vi "Temp_Read_Sub.vi"(0 "VISA Refnum in":refnum<visa-resource-name>, 1 "Setp":refnum<vi>, 2 "Numeric":i32, 3 "String":string, 5 "String to Write":string, 7 "Rate":refnum<vi>, 9 "String to Write 2":string, 11 "Ring Refnum":refnum<vi>, 12 "Ring Refnum 2":refnum<vi>, 13 "String to Write 4":string, 14 "String to Write 3":string) -> (4 "Temp":dbl caption="K" format="%.4g", 6 "dup VISA Session":refnum<visa-resource-name>)   [LabVIEW 2024]
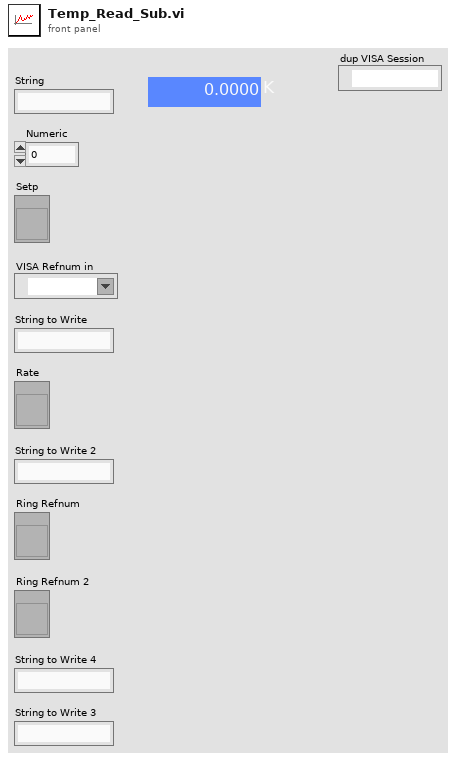
[diagram p1: front panel]
types:
  T1 = enum8{"Enabled", "Disabled", "Disabled and Grayed Out"}
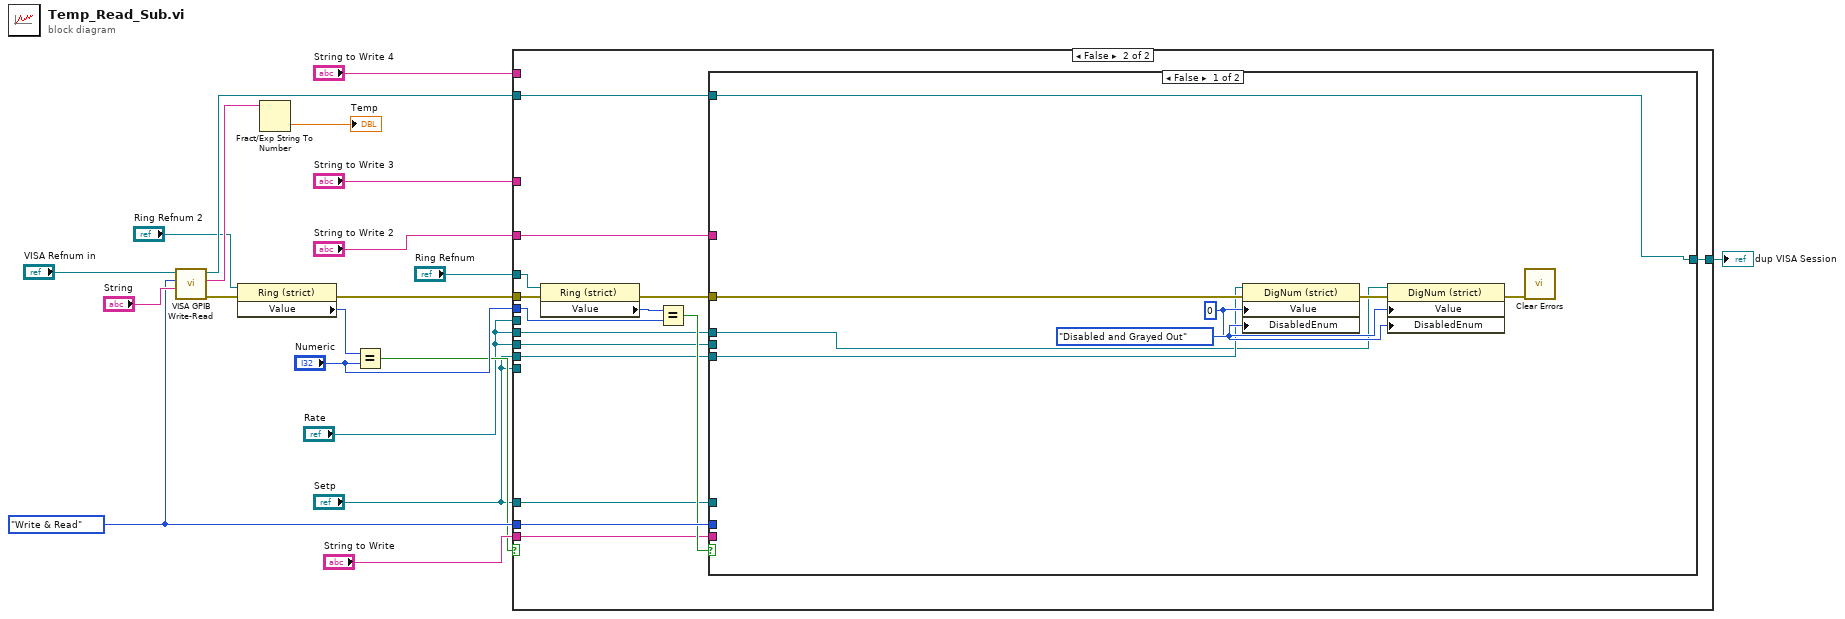
[diagram p0: block diagram]
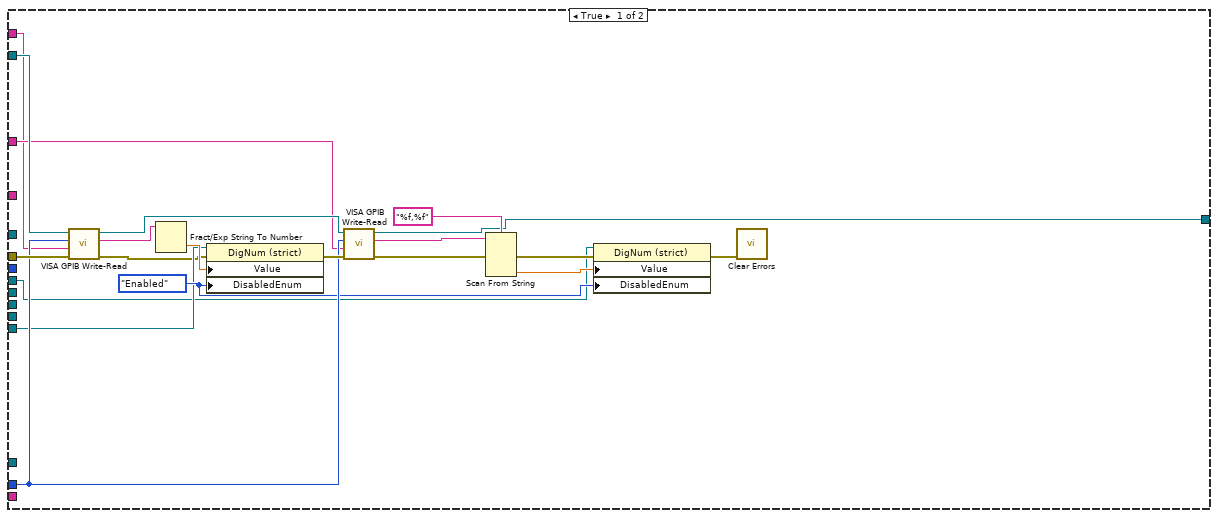
[diagram p2: hidden frame]
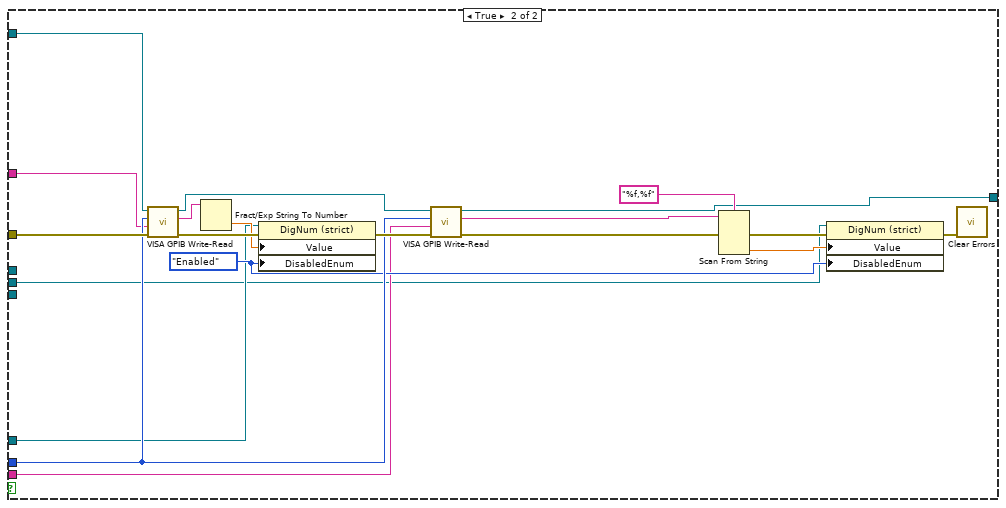
[diagram p3: hidden frame]
diagram:
  w12 = enum16{"Write", "Read", "Write & Read"}."Write & Read" ("Action")
  n1 = call "VISA GPIB Write-Read.vi"("Command"="String", "Action"=w12, "VISA resource name"="VISA Refnum in") -> ("error out"=w9:errorcluster, "String Returned"=w7:string, "dup VISA Session"=w13:refnum<visa-resource-name>)  [unwired: 5 in, 1 out]
  n2 = property on="Property Node" class="Ring (strict)"(reference="Ring Refnum 2", error in=w9) -> (error out=w2:errorcluster, "Value"=w10:u16)  [unwired: 1 out]
  n3 = Fract/Exp String To Number(string=w7) -> (number=→"Temp":dbl)  [unwired: 3 in, 1 out]
  n4 = Equal?(x=w10, y="Numeric") -> (x = y?=w11:bool)
  n5 = case shown="False" w11 {
    tunnel: w2 -> [w40 w53]
    tunnel: w12 -> [w34 w54]
    tunnel: w13 -> [w39 w55]
    tunnel: "Numeric" -> [_ w49]
    tunnel: "String to Write 3" -> [w27 _]
    tunnel: "String to Write 4" -> [w26 _]
    tunnel: "String to Write 2" -> [_ w48]
    tunnel: "String to Write" -> [_ w47]
    tunnel: "Setp" -> [w24 _]
    tunnel: "Rate" -> [w23 _]
    tunnel: "Setp" -> [_ w46]
    tunnel: "Rate" -> [_ w45]
    tunnel: "Setp" -> [_ w44]
    tunnel: "Rate" -> [_ w43]
    tunnel: "Ring Refnum" -> [_ w42]
    tunnel: [w21 w41] -> w1
    frame True {
      w29 = T1."Enabled" ("Disabled")
      n6 = call "VISA GPIB Write-Read.vi"("error in (no error)"=w40, "Command"=w26, "Action"=w34, "VISA resource name"=w39) -> ("error out"=w22:errorcluster, "String Returned"=w38:string, "dup VISA Session"=w35:refnum<visa-resource-name>)  [unwired: 4 in, 1 out]
      n7 = Fract/Exp String To Number(string=w38) -> (number=w37:dbl)  [unwired: 3 in, 1 out]
      n8 = property on="Property Node" class="DigNum (strict)"(reference=w24, error in=w22, "Value"=w37, "DisabledEnum"=w29) -> (error out=w36:errorcluster)  [unwired: 1 out]
      n9 = call "VISA GPIB Write-Read.vi"("error in (no error)"=w36, "Command"=w27, "Action"=w34, "VISA resource name"=w35) -> ("error out"=w33:errorcluster, "String Returned"=w32:string, "dup VISA Session"=w21:refnum<visa-resource-name>)  [unwired: 4 in, 1 out]
      n10 = Scan From String(format string="%f,%f", input string=w32, error in=w33) -> (error out=w30:errorcluster, output 2=w28:dbl)  [unwired: 4 in, 2 out]
      n11 = property on="Property Node" class="DigNum (strict)"(reference=w23, error in=w30, "Value"=w28, "DisabledEnum"=w29) -> (error out=w25:errorcluster)  [unwired: 1 out]
      n12 = call <vilib>:"Clear Errors.vi"("error in (no error)"=w25) -> ()  [unwired: 5 in, 2 out]
    }
    frame False {
      n13 = property on="Property Node" class="Ring (strict)"(reference=w42, error in=w53) -> (error out=w52:errorcluster, "Value"=w51:u16)  [unwired: 1 out]
      n14 = Equal?(x=w51, y=w49) -> (x = y?=w50:bool)
      n15 = case shown="False" w50 {
        tunnel: w52 -> [w63 w83]
        tunnel: w55 -> [w56 w82]
        tunnel: w54 -> [_ w76]
        tunnel: w48 -> [_ w69]
        tunnel: w47 -> [_ w68]
        tunnel: w46 -> [w58 _]
        tunnel: w45 -> [w57 _]
        tunnel: w44 -> [_ w66]
        tunnel: w43 -> [_ w65]
        tunnel: [w56 w64] -> w41
        frame False {
          w61 = T1."Disabled and Grayed Out" ("Disabled")
          w60 = 0
          n16 = property on="Property Node" class="DigNum (strict)"(reference=w58, error in=w63, "Value"=w60, "DisabledEnum"=w61) -> (error out=w62:errorcluster)  [unwired: 1 out]
          n17 = property on="Property Node" class="DigNum (strict)"(reference=w57, error in=w62, "Value"=w60, "DisabledEnum"=w61) -> (error out=w59:errorcluster)  [unwired: 1 out]
          n18 = call <vilib>:"Clear Errors.vi"("error in (no error)"=w59) -> ()  [unwired: 5 in, 2 out]
        }
        frame True {
          w71 = T1."Enabled" ("Disabled")
          n19 = call "VISA GPIB Write-Read.vi"("error in (no error)"=w83, "Command"=w69, "Action"=w76, "VISA resource name"=w82) -> ("error out"=w80:errorcluster, "String Returned"=w81:string, "dup VISA Session"=w77:refnum<visa-resource-name>)  [unwired: 4 in, 1 out]
          n20 = Fract/Exp String To Number(string=w81) -> (number=w79:dbl)  [unwired: 3 in, 1 out]
          n21 = property on="Property Node" class="DigNum (strict)"(reference=w66, error in=w80, "Value"=w79, "DisabledEnum"=w71) -> (error out=w78:errorcluster)  [unwired: 1 out]
          n22 = call "VISA GPIB Write-Read.vi"("error in (no error)"=w78, "Command"=w68, "Action"=w76, "VISA resource name"=w77) -> ("error out"=w75:errorcluster, "String Returned"=w74:string, "dup VISA Session"=w64:refnum<visa-resource-name>)  [unwired: 4 in, 1 out]
          n23 = Scan From String(format string="%f,%f", input string=w74, error in=w75) -> (error out=w72:errorcluster, output 2=w70:dbl)  [unwired: 4 in, 2 out]
          n24 = property on="Property Node" class="DigNum (strict)"(reference=w65, error in=w72, "Value"=w70, "DisabledEnum"=w71) -> (error out=w67:errorcluster)  [unwired: 1 out]
          n25 = call <vilib>:"Clear Errors.vi"("error in (no error)"=w67) -> ()  [unwired: 5 in, 2 out]
        }
      }
    }
  }
  "dup VISA Session" <- w1
